vi "Unhandled state Process.vi"(8 "error in (no error)":errorcluster, 9 "variant":variant, 10 "Unhandled state Case Name":string, 11 "Model in":refnum<class "Model.lvclass">) -> (0 "error out":errorcluster, 3 "Model out":refnum<class "Model.lvclass">)   [LabVIEW 2021, in "Model.lvlib" / "Model.lvclass"]
uses:
  Model.lvclass
  <vilib>/OPCUA/controls/Subscription Data Change.ctl
  <vilib>/OPCUA/controls/NodeId.ctl
  <vilib>/OPCUA/controls/Data Type.ctl
  <vilib>/OPCUA/controls/OPC UA StatusCode.ctl
  Model.lvclass/Model.ctl
  <userlib>/John_Lib/Network_Streams_Connection/NetworkCommand--Cluster.ctl
  6f0a7e90-1539-4457-87b1-6d75e7853941.vi
  <userlib>/John_Lib/AMC_FW/Send Local Message.vi
  <userlib>/John_Lib/AMC_FW/Create Single Message.vi
  <userlib>/John_Lib/AMC_FW/Update Message Routing Info.vi
  <userlib>/John_Lib/AMC_FW/String to Array.vi
  <userlib>/John_Lib/AMC_FW/Send Message.vi
  <userlib>/John_Lib/OPCUA/OPCUA.lvclass
  <userlib>/John_Lib/Network_Streams_Connection/NetworkConnection.lvclass
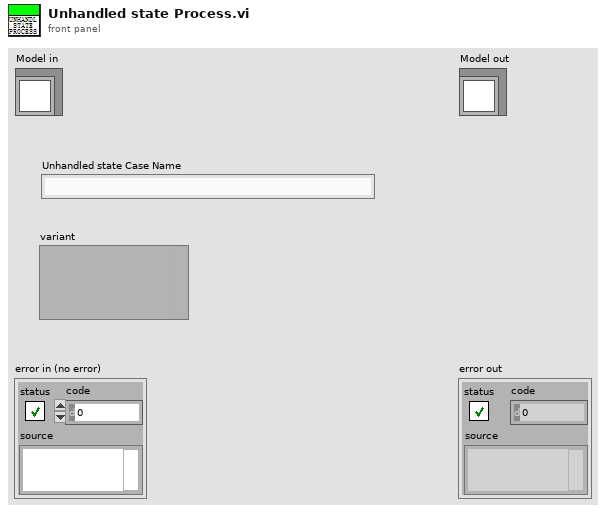
[diagram p1: front panel]
types:
  T1 = typedef "Subscription Data Change.ctl" = cluster{"node ID":T2, " value":variant, "timestamp":timestamp, "data type":T3, "status code":T4}
  T2 = typedef "NodeId.ctl" = string
  T3 = typedef "Data Type.ctl" = u16
  T4 = typedef "OPC UA StatusCode.ctl" = u32
  T5 = typedef "JKI_Network_Streams.lvlib/NetworkConnection.lvclass/NetworkCommand--Cluster.ctl" = cluster{"Command":string, "Arguments":variant, " Msg Id":i32, "Data":string, "Result":string}
  T6 = typedef "Model.lvlib/Model.lvclass/DVR.ctl" = cluster{"JKI_Network_Streams":refnum<class "NetworkConnection.lvclass">, "AMC Q":T7}
  T7 = typedef "Model.lvlib/Model.lvclass/AMC Q.ctl" = cluster{"Main":T8, "OPCUA":T8, "NetworkSteam":T8}
  T8 = typedef "AMC_FW.lvlib/Queue.ctl" = cluster{"Q":T9, "Name":string}
  T9 = typedef "AMC_FW.lvlib/Message Queue.ctl" = refnum<queue>
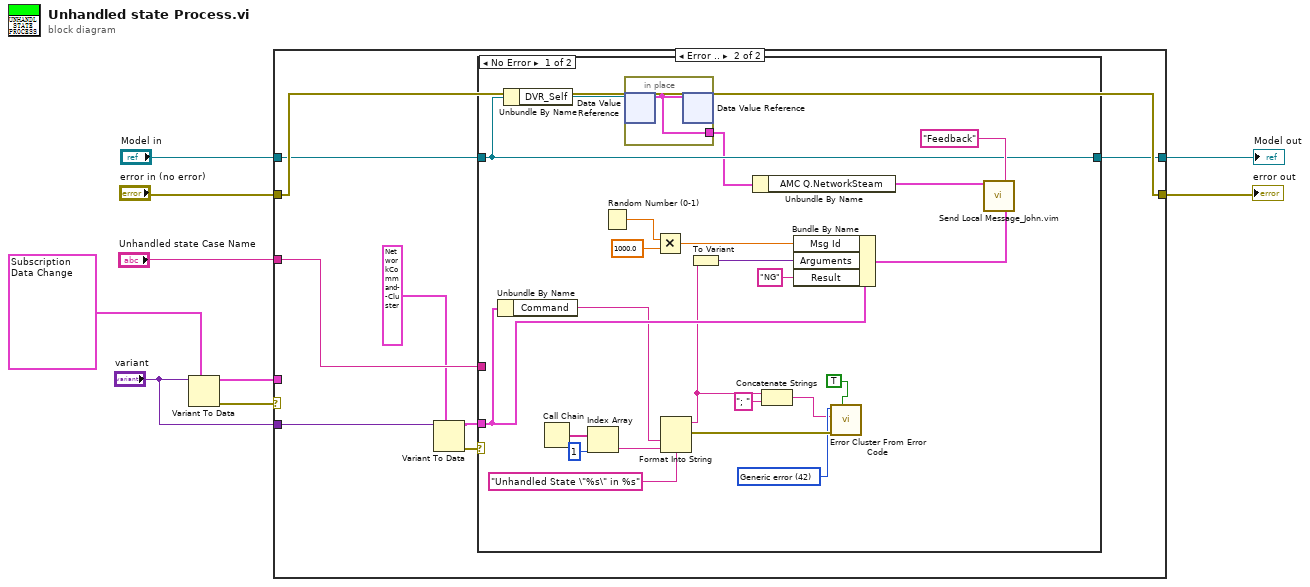
[diagram p0: block diagram]
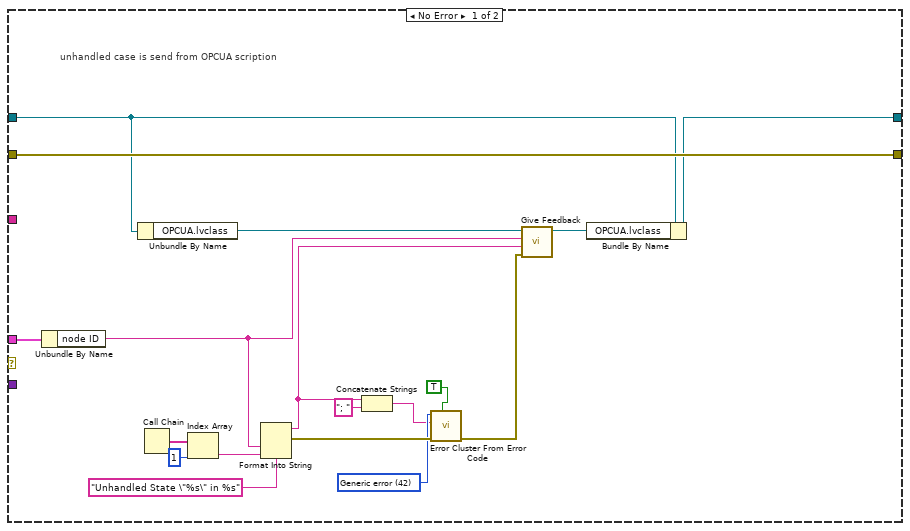
[diagram p2: hidden frame]
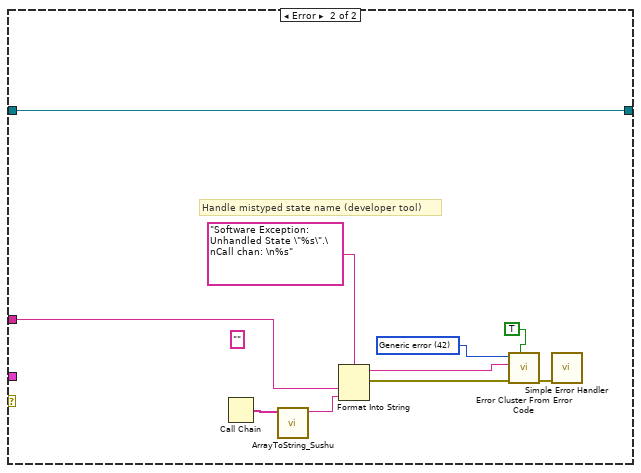
[diagram p3: hidden frame]
diagram:
  n1 = Variant To Data(type=T1 {"node ID"="", " value"=variant, "timestamp"=timestamp(0 s since 1904-01-01), "data type"=1, "status code"=0} ("data change 2"), Variant="variant") -> (data=w2:T1, error out=w8:errorcluster)  [unwired: 1 in]
  n2 = case shown="Error .." w8 {
    tunnel: "Model in" -> [w25 w29]
    tunnel: [w23 w28] -> w6
    tunnel: [w27 w35] -> w5
    tunnel: "error in (no error)" -> [w27 w35]
    tunnel: "Unhandled state Case Name" -> [_ w34]
    tunnel: w2 -> [w26 _]
    tunnel: "variant" -> [_ w33]
    frame No Error {
      w19 = 42 items=["No error", "Argument error", "Memory is full", "Out of zone", "End of file", "File already open", "Generic file I/O error", "File not found", "File permission error", "Disk is full", "Duplicate path", "Too many files open", "System feature not enabled", "Resource file not found", "Cannot add resource", "Resource not found", "Image not found", "Image memory error", "Pen does not exist", "Config type invalid", "Config token not found", "Config parse error", "Config memory error", "Bad external code format", "Bad external code offset", "External code not present", "Null window", "Destroy window error", "Null menu", "Print aborted", "Bad print record", "Print driver error", "Windows error during printing", "Memory error during printing", "Print dialog error", "Generic print error", "Invalid device refnum", "Device not found", "Device parameter error", "Device unit error", "Cannot open device", "Device call aborted", "Generic error", "Cancelled by user", "Object ID too low", "Object ID too high", "Object not in heap", "Unknown heap", "Unknown object (invalid DefProc)", "Unknown object (DefProc not in table)", "Message out of range", "Invalid (null) method", "Unknown message", "Manager call not supported", "Bad address", "Network operation in progress", "Network operation timed out", "Connection is busy", "Network attribute not supported", "Network error", "Address in use", "System out of memory", "Connection aborted", "Connection refused", "Not connected", "Already connected", "Connection closed", "Initialization error (interapplication manager)", "Bad occurrence", "Wait on unbound occurrence handler", "Occurrence queue overflow", "Datalog type conflict", "Unused", "Unrecognized type (interapplication manager)", "Memory corrupt", "Failed to make temporary DLL", "Old CIN version", "Drag socket not found", "Failed to load drop-object", "Failed to register OLE object", "Failed to release OLE object", "Format specifier type mismatch", "Unknown format specifier", "Too few format specifiers", "Too many format specifiers", "Scan failed", "Newer CIN version", "Error converting to variant", "Runtime menu error", "Password tampered", "Variant attribute not found", "Incompatible variant data type", "Event data is not available", "Event Store is not present", "Occurrence is not found", "Event Queue is not created", "Event info is not available", "Refnum passed is NULL", "Error retrieving Class GUID", "Error retrieving CoClass GUID", "Error retrieving TypeLib GUID.", "Bad built application magic bytes.", "Specific driver is different from the specific driver associated with the Logical Name.", "There is no session opened to the class driver.", "Max Error", "MAX - Error with config objects", "MAX - Error loading configuration", "MAX - Group not supported"]
      # "unhandled case is send from OPCUA scription"
      n3 = Unbundle By Name(w26) -> ("node ID"=w15:T2)
      n4 = Unbundle By Name(w25) -> ("OPCUA.lvclass"=w24:refnum<class "OPCUA.lvclass">)
      n5 = Call Chain() -> (call chain=w18:string[])
      n6 = Index Array(array=w18, index=1) -> (element=w16:string)
      n7 = Format Into String(format string="Unhandled State \"%s\" in %s" ("element"), w15, w16) -> (resulting string=w13:string, error out=w21:errorcluster)  [unwired: 2 in]
      n8 = Concatenate Strings(w13, "; " ("string")) -> (w11:string)
      n9 = call <vilib>:"Error Cluster From Error Code.vi"("show call chain? (False)"=TRUE, "error in (no error)"=w21, "error message (\"\")"=w11, "error code (0)"=w19) -> ("error out"=w14:errorcluster)  [unwired: 5 in]
      n10 = call <userlib>:"Give Feedback.vi"("error in (no error)"=w14, "FeedBack Data"=w13, "node ID"=w15, "OPCUA in"=w24) -> ("OPCUA out"=w22:refnum<class "OPCUA.lvclass">)  [unwired: 6 in, 1 out]
      n11 = Bundle By Name(cluster=w25, "OPCUA.lvclass"=w22) -> (w23:refnum<class "Model.lvclass">)
    }
    frame Error {
      n12 = Variant To Data(type=T5 {"Command"="", "Arguments"=variant, " Msg Id"=-1, "Data"="", "Result"=""} ("NetworkCommand"), Variant=w33) -> (data=w30:T5, error out=w31:errorcluster)  [unwired: 1 in]
      n13 = case shown="No Error" w31 {
        tunnel: w34 -> [_ w63]
        tunnel: w30 -> [w48 _]
        tunnel: w29 -> [w38 w60]
        tunnel: [w38 w60] -> w28
        frame No Error {
          w56 = 42 items=["No error", "Argument error", "Memory is full", "Out of zone", "End of file", "File already open", "Generic file I/O error", "File not found", "File permission error", "Disk is full", "Duplicate path", "Too many files open", "System feature not enabled", "Resource file not found", "Cannot add resource", "Resource not found", "Image not found", "Image memory error", "Pen does not exist", "Config type invalid", "Config token not found", "Config parse error", "Config memory error", "Bad external code format", "Bad external code offset", "External code not present", "Null window", "Destroy window error", "Null menu", "Print aborted", "Bad print record", "Print driver error", "Windows error during printing", "Memory error during printing", "Print dialog error", "Generic print error", "Invalid device refnum", "Device not found", "Device parameter error", "Device unit error", "Cannot open device", "Device call aborted", "Generic error", "Cancelled by user", "Object ID too low", "Object ID too high", "Object not in heap", "Unknown heap", "Unknown object (invalid DefProc)", "Unknown object (DefProc not in table)", "Message out of range", "Invalid (null) method", "Unknown message", "Manager call not supported", "Bad address", "Network operation in progress", "Network operation timed out", "Connection is busy", "Network attribute not supported", "Network error", "Address in use", "System out of memory", "Connection aborted", "Connection refused", "Not connected", "Already connected", "Connection closed", "Initialization error (interapplication manager)", "Bad occurrence", "Wait on unbound occurrence handler", "Occurrence queue overflow", "Datalog type conflict", "Unused", "Unrecognized type (interapplication manager)", "Memory corrupt", "Failed to make temporary DLL", "Old CIN version", "Drag socket not found", "Failed to load drop-object", "Failed to register OLE object", "Failed to release OLE object", "Format specifier type mismatch", "Unknown format specifier", "Too few format specifiers", "Too many format specifiers", "Scan failed", "Newer CIN version", "Error converting to variant", "Runtime menu error", "Password tampered", "Variant attribute not found", "Incompatible variant data type", "Event data is not available", "Event Store is not present", "Occurrence is not found", "Event Queue is not created", "Event info is not available", "Refnum passed is NULL", "Error retrieving Class GUID", "Error retrieving CoClass GUID", "Error retrieving TypeLib GUID.", "Bad built application magic bytes.", "Specific driver is different from the specific driver associated with the Logical Name.", "There is no session opened to the class driver.", "Max Error", "MAX - Error with config objects", "MAX - Error loading configuration", "MAX - Group not supported"]
          n14 = Unbundle By Name(w48) -> ("Command"=w47:string)
          n15 = Unbundle By Name(w38) -> ("DVR_Self"=w39:refnum<data-value>)
          n16 = Call Chain() -> (call chain=w55:string[])
          n17 = Index Array(array=w55, index=1) -> (element=w53:string)
          n18 = Random Number (0-1)() -> (number: 0 to 1=w44:dbl)
          n19 = in-place {
            in-place-border: [w59] -> w37
            n20 = in-place-dvr #1(w39) -> (w59:T6)  [unwired: 1 out]
            n21 = in-place-dvr #1(w59) -> ()  [unwired: 2 out]
          }
          n22 = Multiply(x=w44, y=1000.0) -> (x*y=w42:dbl)
          n23 = Format Into String(format string="Unhandled State \"%s\" in %s" ("element"), w47, w53) -> (resulting string=w46:string, error out=w58:errorcluster)  [unwired: 2 in]
          n24 = To Variant(anything=w46) -> (Variant=w45:variant)
          n25 = Unbundle By Name(w37) -> ("AMC Q.NetworkSteam"=w36:T8)
          n26 = Concatenate Strings(w46, "; " ("string")) -> (w51:string)
          n27 = Bundle By Name(cluster=w48, "Msg Id"=w42, "Arguments"=w45, "Result"="NG") -> (w41:T5)
          n28 = call <vilib>:"Error Cluster From Error Code.vi"("show call chain? (False)"=TRUE, "error in (no error)"=w58, "error message (\"\")"=w51, "error code (0)"=w56) -> ()  [unwired: 5 in, 1 out]
          n29 = call "Send Local Message_John.vim"("Queue In"=w36, "Elements in Front"="Feedback", "variant"=w41) -> ()  [unwired: 10 in, 3 out]
        }
        frame Error {
          (unwired) ""
          w65 = 42 items=["No error", "Argument error", "Memory is full", "Out of zone", "End of file", "File already open", "Generic file I/O error", "File not found", "File permission error", "Disk is full", "Duplicate path", "Too many files open", "System feature not enabled", "Resource file not found", "Cannot add resource", "Resource not found", "Image not found", "Image memory error", "Pen does not exist", "Config type invalid", "Config token not found", "Config parse error", "Config memory error", "Bad external code format", "Bad external code offset", "External code not present", "Null window", "Destroy window error", "Null menu", "Print aborted", "Bad print record", "Print driver error", "Windows error during printing", "Memory error during printing", "Print dialog error", "Generic print error", "Invalid device refnum", "Device not found", "Device parameter error", "Device unit error", "Cannot open device", "Device call aborted", "Generic error", "Cancelled by user", "Object ID too low", "Object ID too high", "Object not in heap", "Unknown heap", "Unknown object (invalid DefProc)", "Unknown object (DefProc not in table)", "Message out of range", "Invalid (null) method", "Unknown message", "Manager call not supported", "Bad address", "Network operation in progress", "Network operation timed out", "Connection is busy", "Network attribute not supported", "Network error", "Address in use", "System out of memory", "Connection aborted", "Connection refused", "Not connected", "Already connected", "Connection closed", "Initialization error (interapplication manager)", "Bad occurrence", "Wait on unbound occurrence handler", "Occurrence queue overflow", "Datalog type conflict", "Unused", "Unrecognized type (interapplication manager)", "Memory corrupt", "Failed to make temporary DLL", "Old CIN version", "Drag socket not found", "Failed to load drop-object", "Failed to register OLE object", "Failed to release OLE object", "Format specifier type mismatch", "Unknown format specifier", "Too few format specifiers", "Too many format specifiers", "Scan failed", "Newer CIN version", "Error converting to variant", "Runtime menu error", "Password tampered", "Variant attribute not found", "Incompatible variant data type", "Event data is not available", "Event Store is not present", "Occurrence is not found", "Event Queue is not created", "Event info is not available", "Refnum passed is NULL", "Error retrieving Class GUID", "Error retrieving CoClass GUID", "Error retrieving TypeLib GUID.", "Bad built application magic bytes.", "Specific driver is different from the specific driver associated with the Logical Name.", "There is no session opened to the class driver.", "Max Error", "MAX - Error with config objects", "MAX - Error loading configuration", "MAX - Group not supported"]
          # "Handle mistyped state name (developer tool)"
          n30 = Call Chain() -> (call chain=w62:string[])
          n31 = call <userlib>:"ArrayToString_Sushu.vi"("Array"=w62) -> ("String"=w61:string)  [unwired: 10 in]
          n32 = Format Into String(format string="Software Exception: Unhandled State \"%s\".\nCall chan: \n%s" ("message"), w63, w61) -> (resulting string=w67:string, error out=w69:errorcluster)  [unwired: 2 in]
          n33 = call <vilib>:"Error Cluster From Error Code.vi"("show call chain? (False)"=TRUE, "error in (no error)"=w69, "error message (\"\")"=w67, "error code (0)"=w65) -> ("error out"=w68:errorcluster)  [unwired: 5 in]
          n34 = call <vilib>:"Simple Error Handler.vi"("error in (no error)"=w68) -> ()  [unwired: 4 in, 5 out]
        }
      }
    }
  }
  "error out" <- w5
  "Model out" <- w6
